vi "Configuration parameter reading.vi"(8 "error in (no error)":errorcluster caption="错误输入（无错误）") -> (0 "error out":errorcluster caption="错误输出", 1 "enable":bool, 2 "baud rate (9600)":u32(ring)=4800 caption="波特率" items=["1200"=1200, "2400"=2400, "4800"=4800, "9600"=9600, "19200"=19200, "38400"=38400, "115200"=115200], 3 "VISA resource name":refnum<visa-resource-name> caption="串口", 4 "Shift distance":u32, 5 "电子罗盘":T1={"VISA resource name"="", "baud rate (9600)"=9600, "串口打开"=FALSE} {"baud rate (9600)" items=["1200"=1200, "2400"=2400, "4800"=4800, "9600"=9600, "38400"=38400, "115200"=115200]}, 7 "Calibration angle":sgl)   [LabVIEW 2016, in "AIRMAR WeatherCaster.lvlib"]
uses:
  AIRMAR WeatherCaster.lvlib
  <vilib>/Utility/config.llb/Read Key (String).vi
  <vilib>/Utility/config.llb/Read Key (U32).vi
  <vilib>/Utility/config.llb/Read Key (Boolean).vi
  <vilib>/Utility/config.llb/Read Key (Double).vi
  <vilib>/Utility/config.llb/NI_LVConfig.lvlib
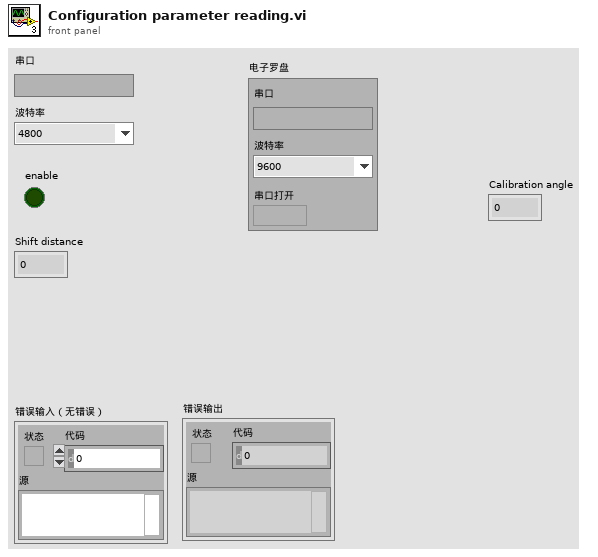
[diagram p1: front panel]
types:
  T1 = cluster{"VISA resource name":refnum<visa-resource-name>, "baud rate (9600)":u32, "串口打开":bool}
  T2 = typedef "NI_LVConfig.lvlib/Config Data RefNum.ctl" = refnum<k1>
  T3 = cluster{"value":string, "value":u32, "value":bool}
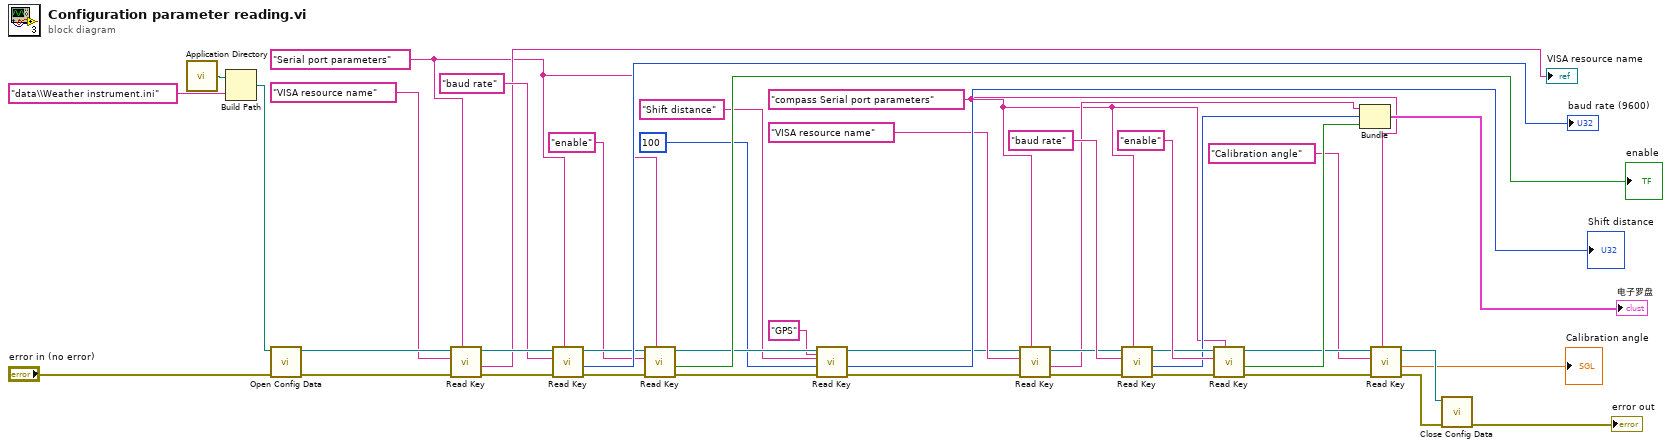
[diagram p0: block diagram]
diagram:
  w3 = "compass Serial port parameters" ("section")
  w29 = "Serial port parameters" ("section")
  n1 = call <vilib>:"Application Directory.vi"() -> ("Application Directory"=w41:path)
  n2 = Build Path(base path=w41, name or relative path="data\\Weather instrument.ini" ("名称或相对路径")) -> (appended path=w42:path)
  n3 = call <vilib>:"Open Config Data.vi"("error in (no error)"="error in (no error)", "configuration file path"=w42) -> ("error out"=w43:errorcluster, "refnum"=w44:T2)  [unwired: 7 in, 1 out]
  n4 = call-poly <vilib>:"Read Key.vi"("section"=w29, "error in (no error)"=w43, "key"="VISA resource name", "refnum"=w44) -> ("error out"=w37:errorcluster, "value"=→"VISA resource name":string, "refnum out"=w38:T2)  [unwired: 4 in, 1 out]
  n5 = call-poly <vilib>:"Read Key.vi"("section"=w29, "error in (no error)"=w37, "key"="baud rate", "refnum"=w38) -> ("error out"=w30:errorcluster, "value"=→"baud rate (9600)":u32, "refnum out"=w31:T2)  [unwired: 4 in, 1 out]
  n6 = call-poly <vilib>:"Read Key.vi"("section"=w29, "error in (no error)"=w30, "key"="enable", "refnum"=w31) -> ("error out"=w25:errorcluster, "value"=→"enable":bool, "refnum out"=w26:T2)  [unwired: 4 in, 1 out]
  n7 = call-poly <vilib>:"Read Key.vi"("section"="GPS", "error in (no error)"=w25, "default value"=u32 100, "key"="Shift distance" ("section"), "refnum"=w26) -> ("error out"=w12:errorcluster, "value"=→"Shift distance":u32, "refnum out"=w13:T2)  [unwired: 3 in, 1 out]
  n8 = call-poly <vilib>:"Read Key.vi"("section"=w3, "error in (no error)"=w12, "key"="VISA resource name", "refnum"=w13) -> ("error out"=w16:errorcluster, "value"=w11:string, "refnum out"=w15:T2)  [unwired: 4 in, 1 out]
  n9 = call-poly <vilib>:"Read Key.vi"("section"=w3, "error in (no error)"=w16, "key"="baud rate", "refnum"=w15) -> ("error out"=w19:errorcluster, "value"=w10:u32, "refnum out"=w18:T2)  [unwired: 4 in, 1 out]
  n10 = call-poly <vilib>:"Read Key.vi"("section"=w3, "error in (no error)"=w19, "key"="enable", "refnum"=w18) -> ("error out"=w5:errorcluster, "value"=w9:bool, "refnum out"=w7:T2)  [unwired: 4 in, 1 out]
  n11 = Bundle("value"=w11, "value"=w10, "value"=w9) -> (→"电子罗盘":T3)  [unwired: 1 in]
  n12 = call-poly <vilib>:"Read Key.vi"("section"=w3, "error in (no error)"=w5, "key"="Calibration angle", "refnum"=w7) -> ("error out"=w4:errorcluster, "value"=→"Calibration angle":dbl, "refnum out"=w6:T2)  [unwired: 4 in, 1 out]
  n13 = call <vilib>:"Close Config Data.vi"("error in (no error)"=w4, "refnum"=w6) -> ("error out"=→"error out":errorcluster)  [unwired: 8 in, 1 out]
